vi "Initialize.vi"(8 "error in":errorcluster, 10 "ID":string, 11 "Client in":refnum<class "Client.lvclass">) -> (0 "error out":errorcluster, 3 "Client out":refnum<class "Client.lvclass">)   [LabVIEW 2014, in "Client.lvclass"]
uses:
  Client.lvclass
  Topic_class/Topic.lvclass
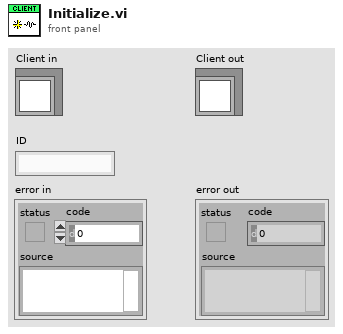
[diagram p1: front panel]
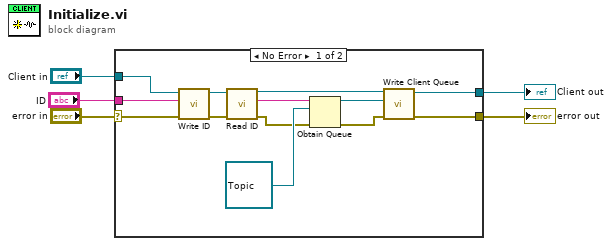
[diagram p0: block diagram]
diagram:
  n1 = case shown="No Error" "error in" {
    selector: "error in" -> [w11 w20]
    tunnel: [w6 w20] -> w4
    tunnel: [w9 w19] -> w2
    tunnel: "Client in" -> [w17 w19]
    tunnel: "ID" -> [w13 _]
    frame No Error {
      n2 = call-dynamic "Write ID.vi"("error in"=w11, "ID"=w13, "Client in"=w17) -> ("error out"=w12:errorcluster, "Client out"=w16:refnum<class "Client.lvclass">)  [unwired: 7 in]
      n3 = call-dynamic "Read ID.vi"("error in"=w12, "Client in"=w16) -> ("error out"=w10:errorcluster, "ID"=w14:string, "Client out"=w15:refnum<class "Client.lvclass">)  [unwired: 7 in]
      n4 = Obtain Queue(name (unnamed)=w14, element data type=refnum<class "Topic.lvclass"> refnum ("Topic.lvclass"), error in (no error)=w10) -> (queue out=w8:refnum<queue>, error out=w7:errorcluster)  [unwired: 2 in, 1 out]
      n5 = call-dynamic "Write Client Queue.vi"("error in"=w7, "Client Queue"=w8, "Client in"=w15) -> ("error out"=w6:errorcluster, "Client out"=w9:refnum<class "Client.lvclass">)  [unwired: 7 in]
    }
    frame Error {
    }
  }
  "error out" <- w4
  "Client out" <- w2
